vi "保存成功对话框 (子VI).vi"(11 "error in (no error)":errorcluster caption="错误输入（无错误）") -> (3 "error out":errorcluster caption="错误输出")   [LabVIEW 2016]
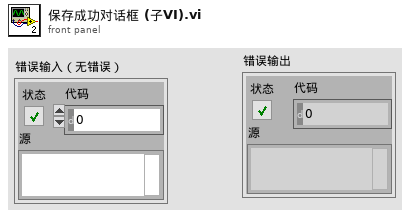
[diagram p1: front panel]
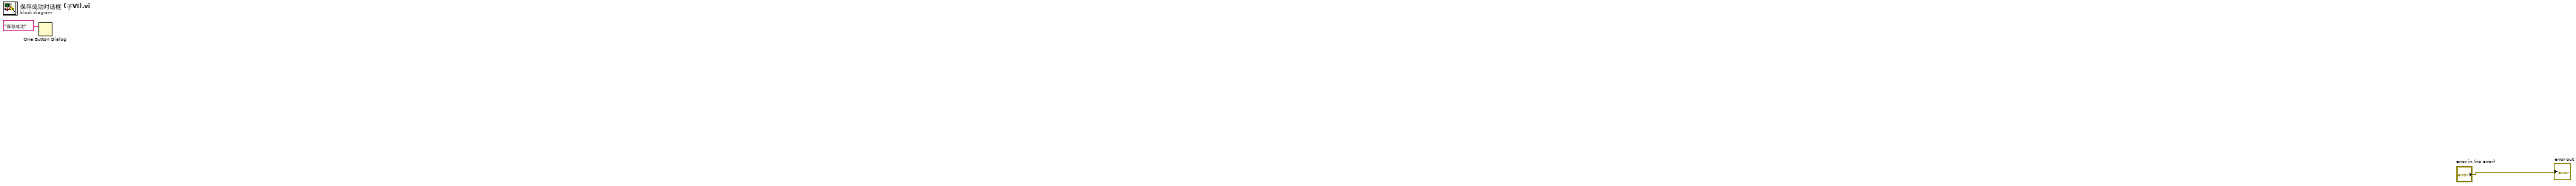
[diagram p0: block diagram]
diagram:
  n1 = One Button Dialog(message="保存成功" ("消息")) -> ()  [unwired: 1 in, 1 out]
  "error out" <- "error in (no error)"
